vi "Ticks to RPM.vi"(8 "Ticks per Rotation":dbl) -> (2 "RPM":dbl)   [LabVIEW 2016]
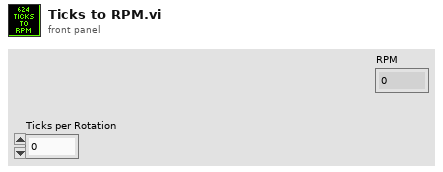
[diagram p1: front panel]
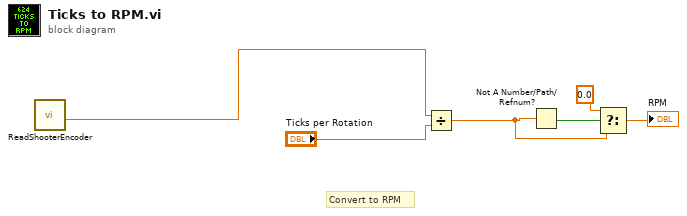
[diagram p0: block diagram]
diagram:
  # "Convert to RPM"
  n1 = call "ReadShooterEncoder.vi"() -> ("TPM"=w1:dbl)  [unwired: 9 in, 2 out]
  n2 = Divide(x=w1, y="Ticks per Rotation") -> (x/y=w3:dbl)
  n3 = Not A Number/Path/Refnum?(number/path/refnum=w3) -> (NaN/Path/Refnum?=w5:bool)
  n4 = Select(t=0.0, s=w5, f=w3) -> (s? t:f=→"RPM":dbl)
